vi "Unpack Request.vi"(11 "Request Data":variant) -> (2 "Is Request":bool, 3 "Data":variant, 4 "Promise":refnum<class "Promise.lvclass">)   [LabVIEW 2020, in "Volatus.lvlib" / "MessageQ.lvclass"]
uses:
  MessageQ.lvclass
  lv-promises/Promises/Promise/Promise.lvclass
  Request Message.ctl
  MessageQ.lvclass/MessageQ.ctl
  Volatus.lvlib
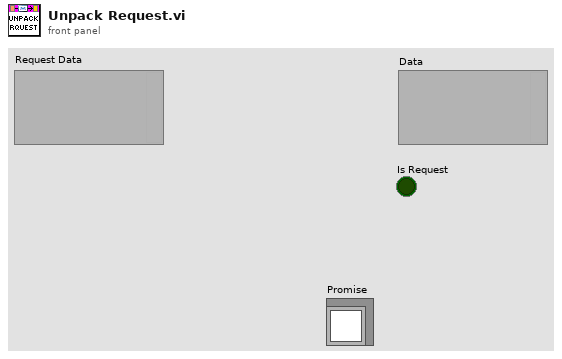
[diagram p1: front panel]
types:
  T1 = typedef "Volatus.lvlib/Request Message.ctl" = cluster{"Promise":refnum<class "Promise.lvclass">, "Data":variant}
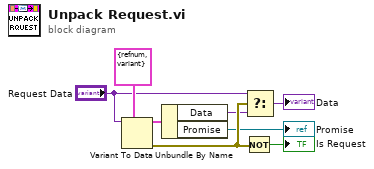
[diagram p0: block diagram]
diagram:
  n1 = Variant To Data(type=T1 {"Promise"=refnum, "Data"=variant} ("Request Message"), Variant="Request Data") -> (data=w6:T1, error out=w8:errorcluster)  [unwired: 1 in]
  n2 = Unbundle By Name(w6) -> ("Data"=w4:variant, "Promise"=→"Promise":refnum<class "Promise.lvclass">)
  n3 = Not(x=w8) -> (.not. x?=→"Is Request":bool)
  n4 = Select(t="Request Data", s=w8, f=w4) -> (s? t:f=→"Data":variant)
